vi "Sample Code.vi"   [LabVIEW 2020]
uses:
  <vilib>/Utility/miscctls.llb/LVFontTypeDef.ctl
  DisplayStyle--enum.ctl
  <vilib>/numeric/Random Number (Range) U64.vi
  <vilib>/numeric/sub_Random U32.vi
  Mensajes.lvlib
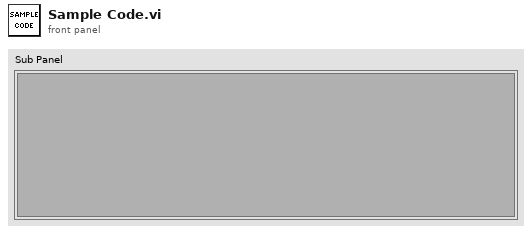
[diagram p1: front panel]
types:
  T1 = typedef "Mensajes.lvlib/DisplayStyle--enum.ctl" = enum16{"Normal", "Backslash", "Password", "Hexadecimal"}
  T2 = typedef "LVFontTypeDef.ctl" = cluster{"Font Name":string, "Size":u16, "Bold":bool, "Italic":bool, "Underline":bool, "Strikeout":bool, "Color":u32}
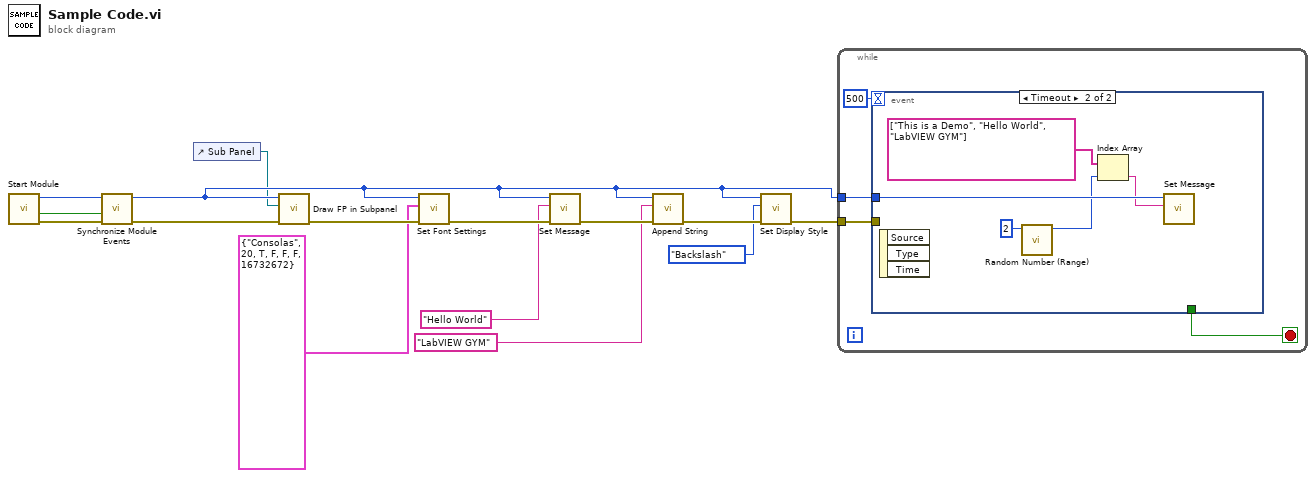
[diagram p0: block diagram]
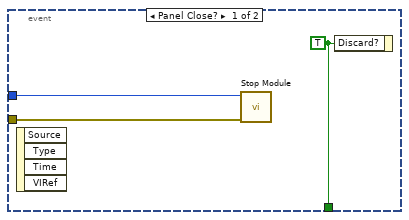
[diagram p2: hidden frame]
diagram:
  n1 = call "Start Module.vi"() -> ("error out"=w15:errorcluster, "Wait for Event Sync?"=w1:bool, "Module ID"=w8:i32)  [unwired: 7 in, 2 out]
  n2 = call "Synchronize Module Events.vi"("error in"=w15, "Wait for Event Sync?"=w1, "Module ID in"=w8) -> ("error out"=w14:errorcluster, "Module ID out"=w7:i32)  [unwired: 7 in]
  n3 = control-ref of="Sub Panel"() -> (w6:refnum<vi>)
  n4 = call "Draw FP in Subpanel.vi"("error in"=w14, "Sub Panel"=w6, "Module ID"=w7) -> ("error out"=w13:errorcluster)  [unwired: 8 in]
  n5 = call "Set Font Settings.vi"("error in"=w13, "Text.Font"=T2 {"Font Name"="Consolas", "Size"=20, "Bold"=TRUE, "Italic"=FALSE, "Underline"=FALSE, "Strikeout"=FALSE, "Color"=16732672}, "Module ID"=w7) -> ("error out"=w12:errorcluster)  [unwired: 8 in]
  n6 = call "Set Message.vi"("error in"=w12, "Message"="Hello World", "Module ID"=w7) -> ("error out"=w11:errorcluster)  [unwired: 8 in]
  n7 = call "Append String.vi"("error in"=w11, "String to Append"="LabVIEW GYM" ("Message"), "Module ID"=w7) -> ("error out"=w10:errorcluster)  [unwired: 8 in]
  n8 = call "Set Display Style.vi"("error in"=w10, "Display Style"=DisplayStyle--enum."Backslash", "Module ID"=w7) -> ("error out"=w9:errorcluster)  [unwired: 8 in]
  n9 = while {
    tunnel: w9 -> [w19]
    tunnel: w7 -> [w18]
    stop <- w17 stop-if-true
    n10 = event shown="[1] Timeout" {
      selector: _ -> [_ _]
      dyn-events: _ -> [_ _]
      timeout: 500 -> [_ _]
      tunnel: w19 -> [w22 _]
      tunnel: w18 -> [w21 w27]
      tunnel: [w20 _] -> w17
      event Panel Close? {
        w20 = TRUE ("Discard?")
        n11 = event-data() -> ()  [unwired: 1 in, 4 out]
        n12 = call "Stop Module.vi"("error in"=w22, "Module ID"=w21) -> ()  [unwired: 9 in, 1 out]
        n13 = event-data("Discard?"=w20) -> ()  [unwired: 1 in, 1 out]
      }
      event Timeout {
        n14 = event-data() -> ()  [unwired: 1 in, 3 out]
        n15 = call-poly <vilib>:"Random Number (Range).vi"("upper bound (100)"=u64 2) -> ("number"=w23:u64)  [unwired: 10 in]
        n16 = Index Array(array=string[] ["This is a Demo", "Hello World", "LabVIEW GYM"], index=w23) -> (element=w25:string)
        n17 = call "Set Message.vi"("Message"=w25, "Module ID"=w27) -> ()  [unwired: 9 in, 1 out]
      }
    }
  }
